vi "Close.vi"(0 "Application Ref":refnum<vi>, 5 "VI Reference Out":refnum<vi>, 11 "error in":errorcluster) -> (15 "error out":errorcluster)   [LabVIEW 2016, in "Drona.lvlib"]
uses:
  Drona.lvlib
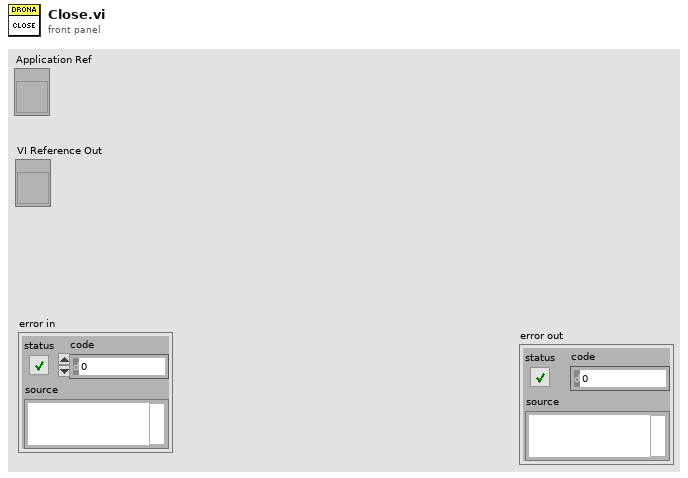
[diagram p1: front panel]
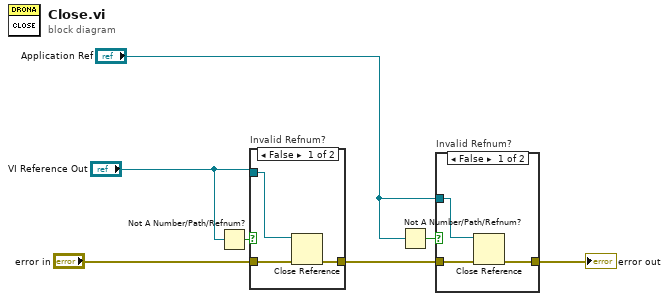
[diagram p0: block diagram]
diagram:
  n1 = Not A Number/Path/Refnum?(number/path/refnum="VI Reference Out") -> (NaN/Path/Refnum?=w4:bool)
  n2 = case "Invalid Refnum?" shown="False" w4 {
    tunnel: "error in" -> [w10 w11]
    tunnel: [w9 w11] -> w7
    tunnel: "VI Reference Out" -> [w8 _]
    frame False {
      n3 = Close Reference(reference=w8, error in (no error)=w10) -> (error out=w9:errorcluster)
    }
    frame True {
    }
  }
  n4 = Not A Number/Path/Refnum?(number/path/refnum="Application Ref") -> (NaN/Path/Refnum?=w2:bool)
  n5 = case "Invalid Refnum?" shown="False" w2 {
    tunnel: w7 -> [w14 w15]
    tunnel: [w13 w15] -> w6
    tunnel: "Application Ref" -> [w12 _]
    frame False {
      n6 = Close Reference(reference=w12, error in (no error)=w14) -> (error out=w13:errorcluster)
    }
    frame True {
    }
  }
  "error out" <- w6
